vi "checkFinishPassTo2ndStrikerPlay.vi"(8 "error in (no error)":errorcluster, 10 "Game":refnum<class "Game.lvclass">, 11 "PassTo2ndStriker in":refnum<class "PassTo2ndStriker.lvclass">) -> (0 "error out":errorcluster, 2 "value":bool, 3 "PassTo2ndStriker out":refnum<class "PassTo2ndStriker.lvclass">)   [LabVIEW 2018, in "PassTo2ndStrikerPlay.lvclass"]
uses:
  PassTo2ndStrikerPlay.lvclass
  temp test/PassTo2ndStriker_class/PassTo2ndStriker.lvclass
  Game_class/Game.lvclass
  Game_class/Game.lvclass/Game.ctl
  Referee_class/Referee.lvclass/Referee.ctl
  Events_class/Events.lvclass/Events.ctl
  Referee_class/command_interpreted.ctl
  Game_class/Read EventsRef.vi
  Events_class/Read touch.vi
  Events_class/Read id_touch.vi
  Events_class/Read ball_out.vi
  Game_class/Read Referee.vi
  Referee_class/Read command_interpreted.vi
  Referee_class/Referee.lvclass
  Events_class/Events.lvclass
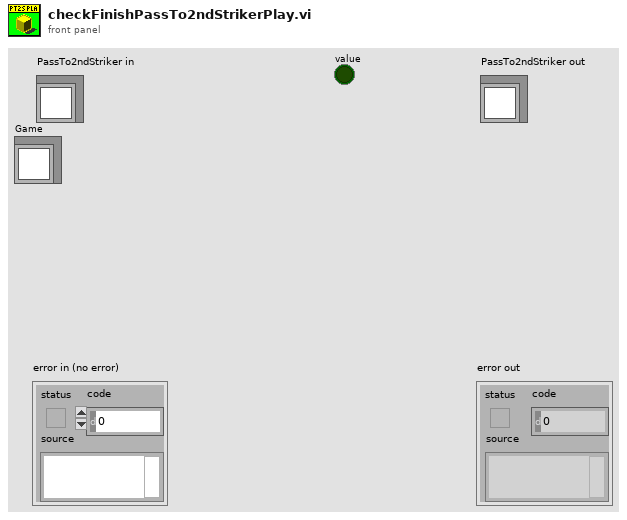
[diagram p1: front panel]
types:
  T1 = typedef "command_interpreted.ctl" = enum16{"Goal Ally", "Goal Enemy", "Ball Placement Enemy", "Ball Placement Ally", "Normal Half Time", "Extra Time  Break", "Extra Half Time", "None", "Post Game", "PKA Normal Start", "Prepare Kickoff Ally", "PKE Normal Start", "Prepare Kickoff Enemy", "Force Start", "Halt", "Timeout", "Prepare Penalty Ally", "Prepare Penalty Enemy", "PPA NormalStart", "PPE Normal Start", "Indirect Free Ally", "Direct Free Enemy", "Direct Free Ally", "Indirect Free Enemy", "Stop"}
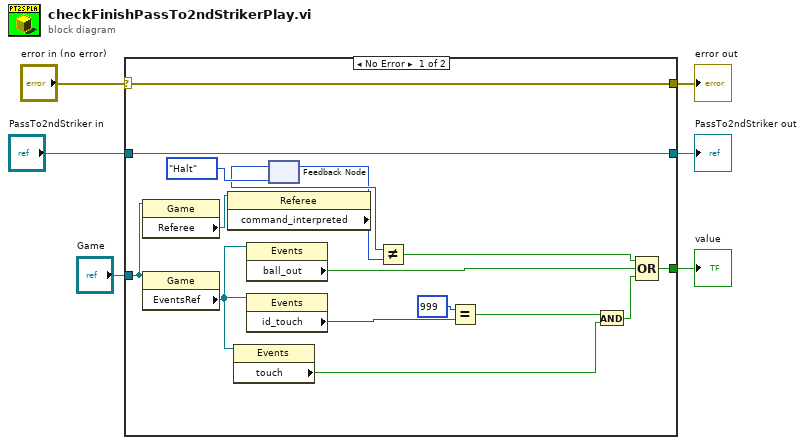
[diagram p0: block diagram]
diagram:
  n1 = case shown="No Error" "error in (no error)" {
    selector: "error in (no error)" -> [w21 w24]
    tunnel: [w21 w24] -> w5
    tunnel: [w22 w23] -> w3
    tunnel: "PassTo2ndStriker in" -> [w22 w23]
    tunnel: [w8 _] -> w2
    tunnel: "Game" -> [w7 _]
    frame No Error {
      n2 = property class="Game"(reference=w7) -> ("Referee"=w14:refnum<class "Referee.lvclass">)  [unwired: 1 in, 2 out]
      n3 = property class="Game"(reference=w7) -> ("EventsRef"=w20:refnum<class "Events.lvclass">)  [unwired: 1 in, 2 out]
      n4 = property class="Referee"(reference=w14) -> ("command_interpreted"=w11:T1)  [unwired: 1 in, 2 out]
      n5 = property class="Events"(reference=w20) -> ("touch"=w9:bool)  [unwired: 1 in, 2 out]
      n6 = property class="Events"(reference=w20) -> ("ball_out"=w17:bool)  [unwired: 1 in, 2 out]
      n7 = property class="Events"(reference=w20) -> ("id_touch"=w18:i32)  [unwired: 1 in, 2 out]
      n8 = feedback #1(command_interpreted."Halt" ("command_interpreted")) -> (w12:T1)
      n9 = feedback-in #1(w11) -> ()
      n10 = Not Equal?(x=w12, y=w11) -> (x != y?=w10:bool)
      n11 = Equal?(x=999 ("id_touch"), y=w18) -> (x = y?=w16:bool)
      n12 = And(x=w16, y=w9) -> (x .and. y?=w15:bool)
      n13 = Compound Arithmetic op=OR(w10, w17, w15) -> (w8:bool)
    }
    frame Error {
    }
  }
  "error out" <- w5
  "PassTo2ndStriker out" <- w3
  "value" <- w2
